vi "BuildReadFrame.vi"(11 "Cmd":string) -> (3 "String":string)   [LabVIEW 2023]
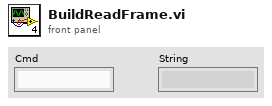
[diagram p1: front panel]
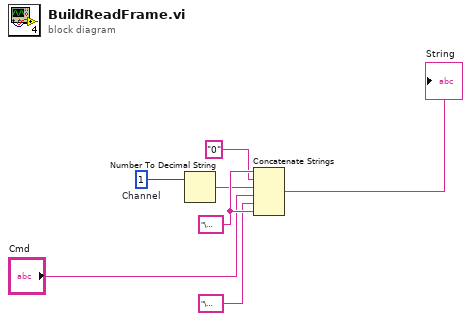
[diagram p0: block diagram]
diagram:
  w6 = "\u0004" ("string")
  w3 = 1  # Channel
  n1 = Number To Decimal String(number=w3) -> (decimal integer string=w2:string)  [unwired: 1 in]
  n2 = Concatenate Strings(w6, "0" ("string"), w2, "Cmd", "\u0005" ("string"), w6) -> (→"String":string)
